vi "get_settings_cluster.vi"(8 "error in (no error)":errorcluster, 11 "DAQ_MG090622Camera in":refnum<class "DAQ_MG090622Camera.lvclass">) -> (0 "error out":errorcluster, 2 "settings cluster":variant, 3 "DAQ_MG090622Camera out":refnum<class "DAQ_MG090622Camera.lvclass">)   [LabVIEW 2010, in "DAQ_MG090622Camera.lvclass"]
uses:
  DAQ_MG090622Camera.lvclass
  DAQ_MG090622Camera.lvclass/DAQ_MG090622Camera.ctl
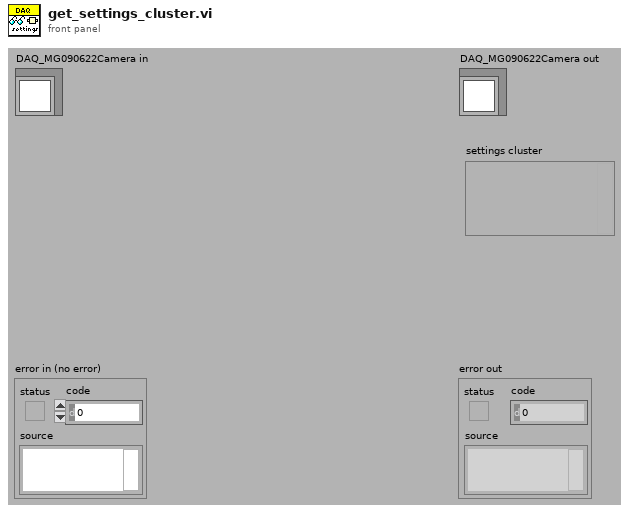
[diagram p1: front panel]
types:
  T1 = typedef "DAQ_MG090622Camera.lvclass/settings_cluster.ctl" = cluster{"duration":dbl[unit]}
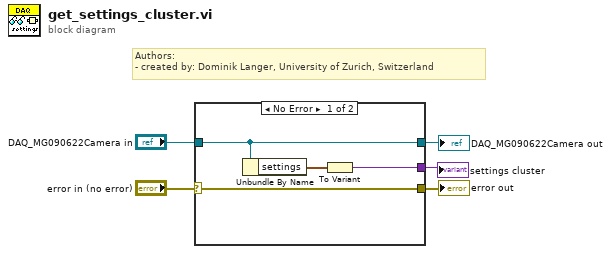
[diagram p0: block diagram]
diagram:
  # "Authors: \n- created by: Dominik Langer, University of Zurich, Switzerland"
  n1 = case shown="No Error" "error in (no error)" {
    selector: "error in (no error)" -> [w6 w10]
    tunnel: "DAQ_MG090622Camera in" -> [w7 w11]
    tunnel: [w8 _] -> w3
    tunnel: [w7 w11] -> w2
    tunnel: [w6 w10] -> w1
    frame No Error {
      n2 = Unbundle By Name(w7) -> ("settings"=w9:T1)
      n3 = To Variant(anything=w9) -> (Variant=w8:variant)
    }
    frame Error {
    }
  }
  "error out" <- w1
  "DAQ_MG090622Camera out" <- w2
  "settings cluster" <- w3
